vi "MCA_count.vi"() -> (0 "多道计数":i32)   [LabVIEW 2014]
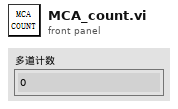
[diagram p1: front panel]
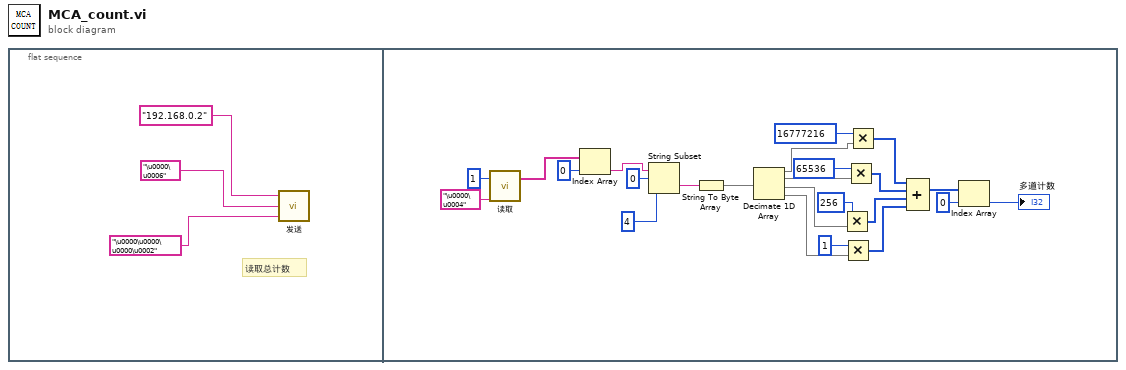
[diagram p0: block diagram]
diagram:
  n1 = flat-sequence {
    frame #0 {
      # "读取总计数"
      n2 = call "发送.vi"("数据（32bit）"="\u0000\u0000\u0000\u0002", "命令(16bit)"="\u0000\u0006", "目标IP"="192.168.0.2") -> ()  [unwired: 1 out]
    }
    frame #1 {
      n3 = call "读取.vi"("命令"="\u0000\u0004", "帧数"=1) -> ("数组"=w25:string[])  [unwired: 1 out]
      n4 = Index Array(array=w25, index=0 ("索引")) -> (element=w23:string)
      n5 = String Subset(string=w23, offset (0)=0 ("偏移量(0)"), length (rest)=4 ("长度（剩余）")) -> (substring=w8:string)
      n6 = String To Byte Array(string=w8) -> (unsigned byte array=w7:u8[])
      n7 = Decimate 1D Array(w7) -> (w9:u8[], w10:u8[], w20:u8[], w19:u8[])
      n8 = Multiply(x=256, y=w20) -> (x*y=w15:i32[])
      n9 = Multiply(x=1, y=w19) -> (x*y=w16:i32[])
      n10 = Multiply(x=65536, y=w10) -> (x*y=w12:i32[])
      n11 = Multiply(x=16777216, y=w9) -> (x*y=w11:i32[])
      n12 = Compound Arithmetic op=ADD(w11, w12, w15, w16) -> (w6:i32[])
      n13 = Index Array(array=w6, index=0 ("索引")) -> (element=→"多道计数":i32)
    }
  }
